vi "LC0-To-Dynamic.vi"(9 "Array":dbl[](array[numeric]), 11 "Waveform":waveform(dbl)) -> (3 "Dynamic Data Type":dynamicdata(waveform))   [LabVIEW 2025]
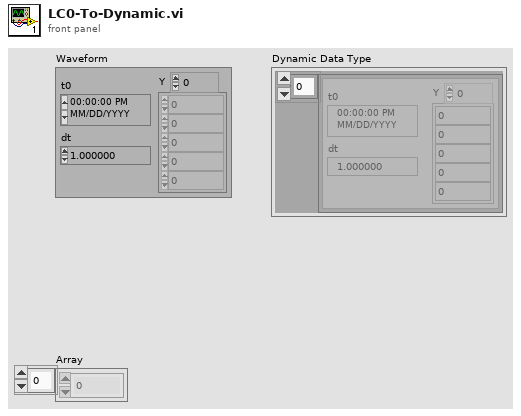
[diagram p1: front panel]
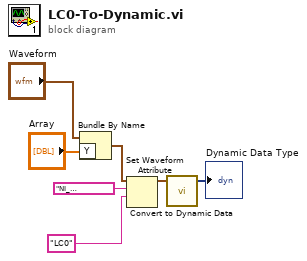
[diagram p0: block diagram]
diagram:
  n1 = Bundle By Name(cluster="Waveform", "Y"="Array") -> (w2:waveform(dbl))
  n2 = Set Waveform Attribute(5:"LC0" ("name"), 6:"NI_ChannelName" ("name"), 7:w2) -> (3:w3:waveform(dbl))  [unwired: 1 in, 2 out]
  n3 = call "Convert to Dynamic Data"("Waveform"=w3) -> ("Dynamic Data Type"=→"Dynamic Data Type":dynamicdata)  [unwired: 3 in]
